vi "Constructor from Excel Sheet.vi"(11 "Excel Sheet.lvclass":refnum<class "Excel Sheet.lvclass">) -> (3 "Data Analyser Report.lvclass":refnum<class "Data Analyser Report.lvclass">)   [LabVIEW 2016, in "Data Analyser Report.lvclass"]
uses:
  Data Analyser Report.lvclass
  Excel Interface/Excel Sheet/Excel Sheet.lvclass
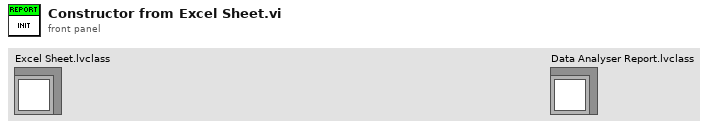
[diagram p1: front panel]
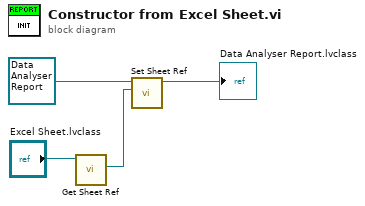
[diagram p0: block diagram]
diagram:
  n1 = call "Get Sheet Ref.vi"("Excel Sheet in"="Excel Sheet.lvclass") -> ("Worksheet"=w2:refnum<k7>)  [unwired: 8 in, 2 out]
  n2 = call-dynamic "Set Sheet Ref.vi"("Worksheet"=w2, "Excel Sheet in"=refnum<class "Data Analyser Report.lvclass"> refnum ("Data Analyser Report.lvclass")) -> ("Excel Sheet out"=→"Data Analyser Report.lvclass":refnum<class "Data Analyser Report.lvclass">)  [unwired: 8 in, 1 out]
